vi "Initialize.vi"(11 "Self Actor in":refnum<class "Self Actor.lvclass">) -> (0 "error out":errorcluster, 3 "Self Actor out":refnum<class "Self Actor.lvclass">)   [LabVIEW 2021, in "AAM.lvlib" / "Self Actor.lvclass"]
uses:
  Self Actor.lvclass
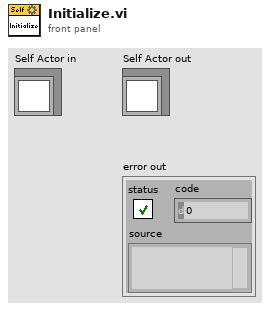
[diagram p1: front panel]
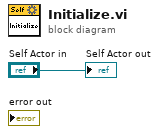
[diagram p0: block diagram]
diagram:
  "Self Actor out" <- "Self Actor in"
